vi "MNIST_data_txt_to_csv.vi"() -> ()   [LabVIEW 2021]
uses:
  <vilib>/Utility/file.llb/Read Delimited Spreadsheet (DBL).vi
  <vilib>/Utility/file.llb/Write Delimited Spreadsheet (DBL).vi
panel:
  out "size(s)":i32[](array[numeric])
  out "subarray":dbl[][](array[numeric])
  out "Intensity Graph":dbl[][](graph)
  in  "file path (dialog if empty) 2":path
  out "all rows":dbl[][](array[numeric])
  in  "file path (dialog if empty)":path
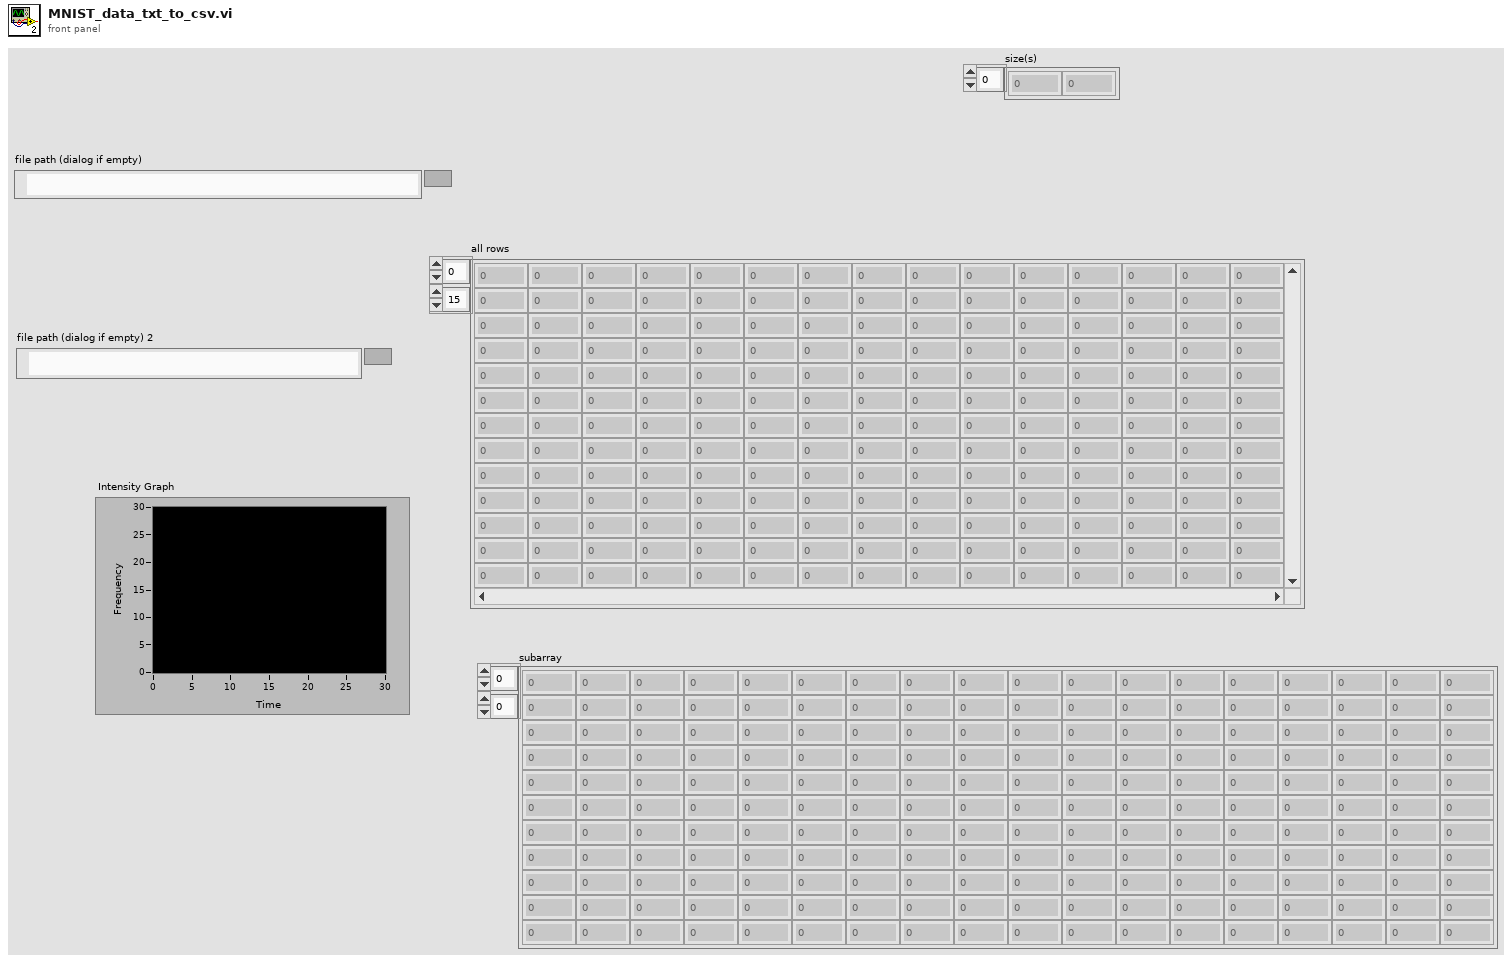
[diagram p1: front panel]
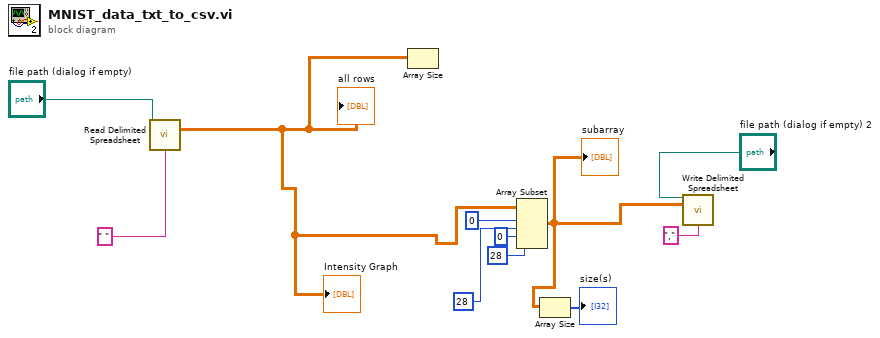
[diagram p0: block diagram]
diagram:
  n1 = call-poly <vilib>:"Read Delimited Spreadsheet.vi"("file path (dialog if empty)"="file path (dialog if empty)", "delimiter (\\t)"=" " ("delimiter (\\t)")) -> ("all rows"=w7:dbl[][])  [unwired: 8 in, 5 out]
  "all rows" <- w7
  "Intensity Graph" <- w7
  n2 = Array Size(array=w7) -> ()  [unwired: 1 out]
  n3 = Array Subset(array=w7, index (row)=0 ("index"), length (row)=28 ("length"), index (col)=0 ("index"), length (col)=28 ("length")) -> (w1:dbl[][])
  "subarray" <- w1
  n4 = Array Size(array=w1) -> (size(s)=→"size(s)":i32[])
  n5 = call-poly <vilib>:"Write Delimited Spreadsheet.vi"("file path (dialog if empty)"="file path (dialog if empty) 2", "2D data"=w1, "delimiter (\\t)"="," ("delimiter (\\t)")) -> ()  [unwired: 11 in, 2 out]
